vi "add_lookup_event_listener.vi"(8 "error in (no error)":errorcluster, 9 "Lookup Listener User Event":refnum<user-event>, 10 "Base Class (LabVIEW Object)":refnum<class>, 11 "Default Lookup in":refnum<class "Default Lookup.lvclass">) -> (0 "error out":errorcluster, 3 "Default Lookup out":refnum<class "Default Lookup.lvclass">)   [LabVIEW 2019, in "Default Lookup.lvclass"]
uses:
  Default Lookup.lvclass
  Default Lookup.lvclass/Default Lookup.ctl
  types/lookup_data.ctl
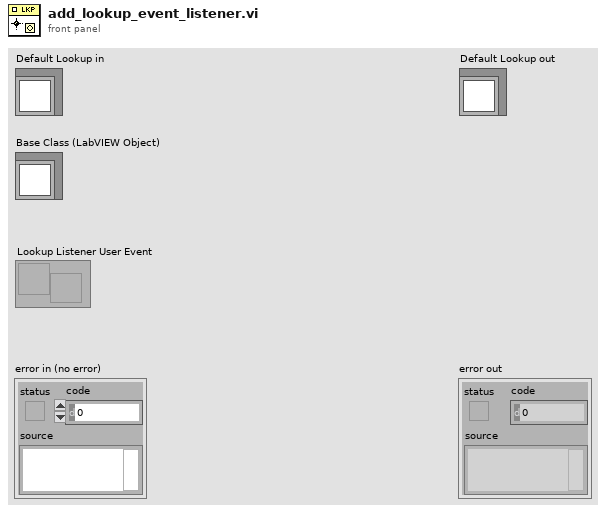
[diagram p1: front panel]
types:
  T1 = typedef "Default Lookup.lvclass/lookup_data.ctl" = cluster{"instances":refnum<data-value>[], "listeners":refnum<user-event>[]}
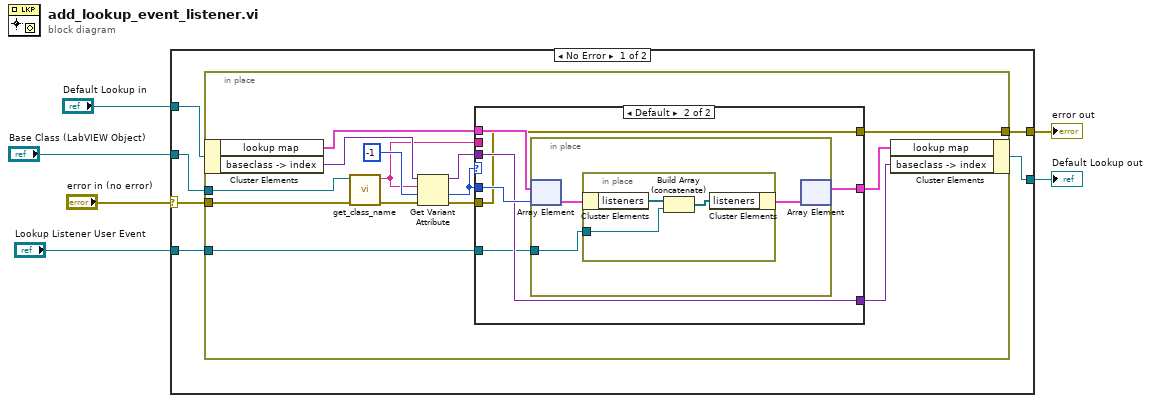
[diagram p0: block diagram]
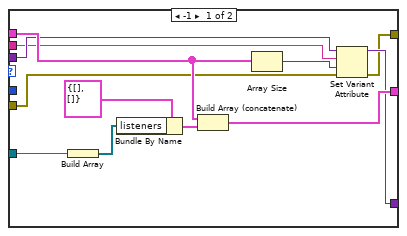
[diagram p2: hidden frame]
diagram:
  n1 = case shown="No Error" "error in (no error)" {
    selector: "error in (no error)" -> [w11 w51]
    tunnel: "Default Lookup in" -> [w12 w52]
    tunnel: "Base Class (LabVIEW Object)" -> [w8 _]
    tunnel: [w10 w52] -> w2
    tunnel: [w9 w51] -> w4
    tunnel: "Lookup Listener User Event" -> [w7 _]
    frame No Error {
      n2 = in-place {
        in-place-border: w8 -> [w25]
        in-place-border: w11 -> [w24]
        in-place-border: [w14] -> w9
        in-place-border: w7 -> [w13]
        n3 = in-place-cluster #1(w12) -> ("lookup map"=w21:T1[], "baseclass -> index"=w26:variant)
        n4 = call "get_class_name.vi"("error in (no error)"=w24, "LabVIEW Object in"=w25) -> ("error out"=w23:errorcluster, "class name"=w18:string)  [unwired: 8 in]
        n5 = Get Variant Attribute(Variant=w26, name=w18, default value (empty Variant)=-1, error in=w23) -> (duplicate Variant=w19:variant, value=w15:i32, error out=w17:errorcluster)  [unwired: 1 out]
        n6 = case shown="Default" w15 {
          tunnel: w21 -> [w35 w44]
          tunnel: [w36 w43] -> w20
          tunnel: w19 -> [w34 w41]
          tunnel: w18 -> [w33 _]
          tunnel: w17 -> [w31 w40]
          tunnel: [w30 w41] -> w16
          tunnel: w15 -> [_ w42]
          tunnel: [w29 w40] -> w14
          tunnel: w13 -> [w28 w39]
          frame -1 {
            n7 = Build Array(w28) -> (w27:refnum<user-event>[])
            n8 = Bundle By Name(cluster=T1 {"instances"=[], "listeners"=[]} ("lookup data"), "listeners"=w27) -> (w37:T1)
            n9 = Build Array (concatenate)(w35, w37) -> (w36:T1[])
            n10 = Array Size(array=w35) -> (size(s)=w32:i32)
            n11 = Set Variant Attribute(Variant=w34, name=w33, value=w32, error in=w31) -> (Variant out=w30:variant, error out=w29:errorcluster)  [unwired: 1 out]
          }
          frame Default {
            n12 = in-place {
              in-place-border: w39 -> [w45]
              n13 = in-place-array #2(w44, w42) -> (w47:T1)
              n14 = in-place {
                in-place-border: w45 -> [w48]
                n15 = in-place-cluster #3(w47) -> ("listeners"=w50:refnum<user-event>[])
                n16 = Build Array (concatenate)(w50, w48) -> (w49:refnum<user-event>[])
                n17 = in-place-cluster #3("listeners"=w49) -> (w46:T1)
              }
              n18 = in-place-array #2(w46) -> (w43:T1[])  [unwired: 1 out]
            }
          }
        }
        n19 = in-place-cluster #1("lookup map"=w20, "baseclass -> index"=w16) -> (w10:refnum<class "Default Lookup.lvclass">)
      }
    }
    frame Error {
    }
  }
  "error out" <- w4
  "Default Lookup out" <- w2
